vi "NF LI56xx VI Tree.vi"   [LabVIEW 2019]
doc: "The VI Tree displays all the user-callable VIs of the instrument driver in an organized table."
panel:
  # "Copyright(c) 2019 NF Corporation All rights reserved."
  # "SEE DIAGRAM\nFOR VI TREE."
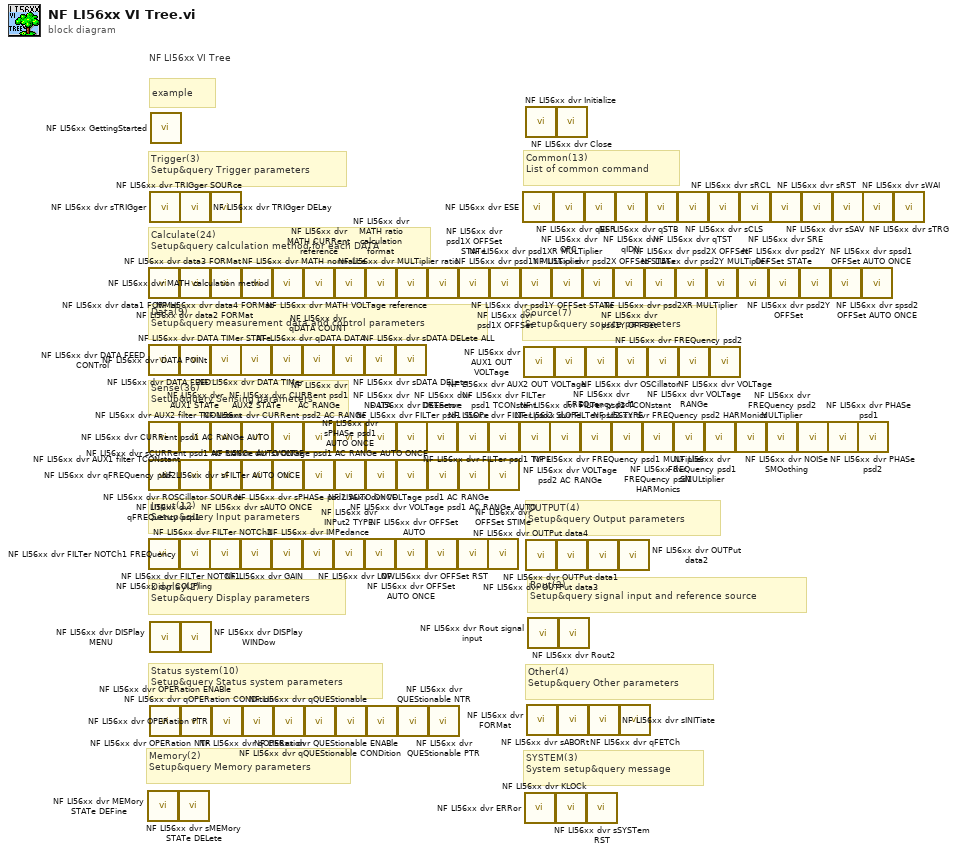
[diagram p0: block diagram]
diagram:
  # "Source(7)\nSetup&query source parameters"
  # "Common(13)\nList of common command"
  # "SYSTEM(3)\nSystem setup&query message"
  # "Memory(2)\nSetup&query Memory parameters"
  # "Status system(10)\nSetup&query Status system parameters"
  # "Other(4)\nSetup&query Other parameters"
  # "OUTPUT(4)\nSetup&query Output parameters"
  # "Input(12)\nSetup&query Input parameters"
  # "Sense(36)\nSetup&query Sensing parameters"
  # "NF LI56xx VI Tree"
  # "Display(2)\nSetup&query Display parameters"
  # "Rout(2)\nSetup&query signal input and reference source"
  # "Calculate(24)\nSetup&query calculation method for each DATA"
  # "Trigger(3)\nSetup&query Trigger parameters"
  # "Data(9)\nSetup&query measurement data and control parameters"
  # "example"
  n1 = call "NF LI56xx dvr MEMory STATe DEFine.vi"() -> ()  [unwired: 9 in, 3 out]
  n2 = call "NF LI56xx dvr data1 FORMat.vi"() -> ()  [unwired: 9 in, 3 out]
  n3 = call "NF LI56xx dvr DATA FEED CONTrol.vi"() -> ()  [unwired: 9 in, 3 out]
  n4 = call "NF LI56xx dvr AUX1 filter TCONstant.vi"() -> ()  [unwired: 9 in, 3 out]
  n5 = call "NF LI56xx dvr qFREQuency psd1.vi"() -> ()  [unwired: 9 in, 3 out]
  n6 = call "NF LI56xx dvr COUPling.vi"() -> ("error out"=w13:errorcluster, "VISA resource name copy"=w12:refnum<visa-resource-name>)  [unwired: 9 in, 1 out]
  n7 = call "NF LI56xx dvr sTRIGger.vi"() -> ("error out"=w4:errorcluster, "VISA resource name copy"=w3:refnum<visa-resource-name>)  [unwired: 10 in]
  n8 = call "NF LI56xx dvr DISPlay MENU.vi"() -> ()  [unwired: 9 in, 3 out]
  n9 = call "NF LI56xx dvr OPERation ENABle.vi"() -> ()  [unwired: 9 in, 3 out]
  n10 = call "NF LI56xx GettingStarted.vi"() -> ()  [unwired: 12 in]
  n11 = call "NF LI56xx dvr sMEMory STATe DELete.vi"() -> ()  [unwired: 10 in, 2 out]
  n12 = call "NF LI56xx dvr TRIGger DELay.vi"() -> ()  [unwired: 9 in, 3 out]
  n13 = call "NF LI56xx dvr data2 FORMat.vi"() -> ()  [unwired: 9 in, 3 out]
  n14 = call "NF LI56xx dvr DATA FEED.vi"() -> ("error out"=w32:errorcluster, "VISA resource name copy"=w31:refnum<visa-resource-name>)  [unwired: 9 in, 1 out]
  n15 = call "NF LI56xx dvr AUX1 STATe.vi"() -> ()  [unwired: 9 in, 3 out]
  n16 = call "NF LI56xx dvr qFREQuency psd2.vi"() -> ()  [unwired: 9 in, 3 out]
  n17 = call "NF LI56xx dvr FILTer NOTCh1 FREQuency.vi"() -> ()  [unwired: 9 in, 3 out]
  n18 = call "NF LI56xx dvr DISPlay WINDow.vi"() -> ()  [unwired: 9 in, 3 out]
  n19 = call "NF LI56xx dvr OPERation NTR.vi"() -> ()  [unwired: 9 in, 3 out]
  n20 = call "NF LI56xx dvr FILTer NOTCh1.vi"("error in"=w13, "VISA resource name"=w12) -> ("error out"=w11:errorcluster, "query notch filter enable"=w10:bool, "VISA resource name copy"=w9:refnum<visa-resource-name>)  [unwired: 7 in]
  n21 = call "NF LI56xx dvr TRIGger SOURce.vi"("error in"=w4, "VISA resource name"=w3) -> ()  [unwired: 7 in, 3 out]
  n22 = call "NF LI56xx dvr data3 FORMat.vi"() -> ()  [unwired: 9 in, 3 out]
  n23 = call "NF LI56xx dvr DATA POINt.vi"() -> ()  [unwired: 9 in, 3 out]
  n24 = call "NF LI56xx dvr AUX2 filter TCONstant.vi"() -> ()  [unwired: 9 in, 3 out]
  n25 = call "NF LI56xx dvr ROSCillator SOURce.vi"() -> ("error out"=w15:errorcluster, "VISA resource name copy"=w14:refnum<visa-resource-name>)  [unwired: 9 in, 1 out]
  n26 = call "NF LI56xx dvr OPERation PTR.vi"() -> ()  [unwired: 9 in, 3 out]
  n27 = call "NF LI56xx dvr DATA TIMer STATe.vi"("error in"=w32, "VISA resource name"=w31) -> ()  [unwired: 7 in, 3 out]
  n28 = call "NF LI56xx dvr FILTer NOTCh2.vi"() -> ()  [unwired: 9 in, 3 out]
  n29 = call "NF LI56xx dvr data4 FORMat.vi"() -> ()  [unwired: 9 in, 3 out]
  n30 = call "NF LI56xx dvr AUX2 STATe.vi"() -> ()  [unwired: 9 in, 3 out]
  n31 = call "NF LI56xx dvr sAUTO ONCE.vi"() -> ()  [unwired: 10 in, 2 out]
  n32 = call "NF LI56xx dvr qOPERation CONDition.vi"() -> ()  [unwired: 9 in, 3 out]
  n33 = call "NF LI56xx dvr DATA TIMer.vi"() -> ()  [unwired: 9 in, 3 out]
  n34 = call "NF LI56xx dvr GAIN.vi"("error in"=w11, "Read(F)"=w10, "VISA resource name"=w9) -> ()  [unwired: 6 in, 3 out]
  n35 = call "NF LI56xx dvr MATH calculation method.vi"() -> ()  [unwired: 9 in, 3 out]
  n36 = call "NF LI56xx dvr CURRent psd1 AC RANGe AUTO.vi"() -> ()  [unwired: 9 in, 3 out]
  n37 = call "NF LI56xx dvr sCURRent psd1 AC RANGe AUTO ONCE.vi"("error in"=w15, "VISA resource name"=w14) -> ()  [unwired: 8 in, 2 out]
  n38 = call "NF LI56xx dvr qOPERation.vi"() -> ()  [unwired: 9 in, 3 out]
  n39 = call "NF LI56xx dvr qDATA COUNT.vi"() -> ()  [unwired: 9 in, 3 out]
  n40 = call "NF LI56xx dvr IMPedance.vi"() -> ()  [unwired: 9 in, 3 out]
  n41 = call "NF LI56xx dvr MATH CURRent reference.vi"() -> ()  [unwired: 9 in, 3 out]
  n42 = call "NF LI56xx dvr CURRent psd1 AC RANGe.vi"() -> ()  [unwired: 9 in, 3 out]
  n43 = call "NF LI56xx dvr sFILTer AUTO ONCE.vi"() -> ()  [unwired: 10 in, 2 out]
  n44 = call "NF LI56xx dvr qQUEStionable CONDition.vi"() -> ()  [unwired: 9 in, 3 out]
  n45 = call "NF LI56xx dvr qDATA DATA.vi"() -> ()  [unwired: 10 in, 2 out]
  n46 = call "NF LI56xx dvr INPut2 TYPE.vi"() -> ()  [unwired: 9 in, 3 out]
  n47 = call "NF LI56xx dvr MATH normalize.vi"() -> ()  [unwired: 9 in, 3 out]
  n48 = call "NF LI56xx dvr CURRent psd2 AC RANGe.vi"() -> ()  [unwired: 9 in, 3 out]
  n49 = call "NF LI56xx dvr sPHASe psd1 AUTO ONCE.vi"() -> ()  [unwired: 10 in, 2 out]
  n50 = call "NF LI56xx dvr qQUEStionable.vi"() -> ()  [unwired: 9 in, 3 out]
  n51 = call "NF LI56xx dvr sDATA DELete ALL.vi"() -> ()  [unwired: 10 in, 2 out]
  n52 = call "NF LI56xx dvr LOW.vi"() -> ()  [unwired: 9 in, 3 out]
  n53 = call "NF LI56xx dvr MATH ratio calculation format.vi"() -> ()  [unwired: 9 in, 3 out]
  n54 = call "NF LI56xx dvr DATA.vi"() -> ("error out"=w30:errorcluster, "VISA resource name copy"=w29:refnum<visa-resource-name>)  [unwired: 9 in, 1 out]
  n55 = call "NF LI56xx dvr sPHASe psd2 AUTO ONCE.vi"() -> ()  [unwired: 10 in, 2 out]
  n56 = call "NF LI56xx dvr QUEStionable ENABle.vi"() -> ()  [unwired: 9 in, 3 out]
  n57 = call "NF LI56xx dvr sDATA DELete.vi"() -> ()  [unwired: 10 in, 2 out]
  n58 = call "NF LI56xx dvr OFFSet AUTO ONCE.vi"() -> ()  [unwired: 10 in, 2 out]
  n59 = call "NF LI56xx dvr MATH VOLTage reference.vi"() -> ()  [unwired: 9 in, 3 out]
  n60 = call "NF LI56xx dvr DETector.vi"() -> ("error out"=w28:errorcluster, "VISA resource name copy"=w27:refnum<visa-resource-name>)  [unwired: 9 in, 1 out]
  n61 = call "NF LI56xx dvr sVOLTage psd1 AC RANGe AUTO ONCE.vi"() -> ()  [unwired: 10 in, 2 out]
  n62 = call "NF LI56xx dvr QUEStionable NTR.vi"() -> ()  [unwired: 9 in, 3 out]
  n63 = call "NF LI56xx dvr DREServe.vi"("error in"=w30, "VISA resource name"=w29) -> ()  [unwired: 7 in, 3 out]
  n64 = call "NF LI56xx dvr OFFSet AUTO.vi"() -> ()  [unwired: 9 in, 3 out]
  n65 = call "NF LI56xx dvr MULTiplier ratio.vi"() -> ()  [unwired: 9 in, 3 out]
  n66 = call "NF LI56xx dvr VOLTage psd1 AC RANGe AUTO.vi"() -> ("error out"=w18:errorcluster, "query AC range \nauto"=w17:bool, "VISA resource name copy"=w16:refnum<visa-resource-name>)  [unwired: 9 in]
  n67 = call "NF LI56xx dvr QUEStionable PTR.vi"() -> ()  [unwired: 9 in, 3 out]
  n68 = call "NF LI56xx dvr FILTer psd1 SLOPe.vi"("error in"=w28, "VISA resource name"=w27) -> ()  [unwired: 7 in, 3 out]
  n69 = call "NF LI56xx dvr OFFSet RST.vi"() -> ()  [unwired: 10 in, 2 out]
  n70 = call "NF LI56xx dvr psd1X OFFSet STATe.vi"() -> ()  [unwired: 9 in, 3 out]
  n71 = call "NF LI56xx dvr VOLTage psd1 AC RANGe.vi"() -> ()  [unwired: 9 in, 3 out]
  n72 = call "NF LI56xx dvr OFFSet STIMe.vi"() -> ()  [unwired: 9 in, 3 out]
  n73 = call "NF LI56xx dvr FILTer psd1 TCONstant.vi"() -> ("error out"=w26:errorcluster, "VISA resource name copy"=w25:refnum<visa-resource-name>)  [unwired: 9 in, 1 out]
  n74 = call "NF LI56xx dvr VOLTage psd2 AC RANGe.vi"("error in"=w18, "Read(F)"=w17, "VISA resource name"=w16) -> ()  [unwired: 6 in, 3 out]
  n75 = call "NF LI56xx dvr psd1X OFFSet.vi"() -> ()  [unwired: 9 in, 3 out]
  n76 = call "NF LI56xx dvr FILTer psd1 TYPE.vi"() -> ("error out"=w24:errorcluster, "VISA resource name copy"=w23:refnum<visa-resource-name>)  [unwired: 9 in, 1 out]
  n77 = call "NF LI56xx dvr psd1XR MULTiplier.vi"() -> ()  [unwired: 9 in, 3 out]
  n78 = call "NF LI56xx dvr ESE.vi"() -> ()  [unwired: 9 in, 3 out]
  n79 = call "NF LI56xx dvr AUX1 OUT VOLTage.vi"() -> ()  [unwired: 9 in, 3 out]
  n80 = call "NF LI56xx dvr ERRor.vi"() -> ()  [unwired: 12 in, 4 out]
  n81 = call "NF LI56xx dvr Initialize.vi"() -> ()  [unwired: 9 in, 3 out]
  n82 = call "NF LI56xx dvr OUTPut data3.vi"() -> ()  [unwired: 9 in, 3 out]
  n83 = call "NF LI56xx dvr FORMat.vi"() -> ()  [unwired: 9 in, 3 out]
  n84 = call "NF LI56xx dvr Rout signal input.vi"() -> ()  [unwired: 9 in, 3 out]
  n85 = call "NF LI56xx dvr FILTer psd2 SLOPe.vi"("error in"=w26, "VISA resource name"=w25) -> ()  [unwired: 7 in, 3 out]
  n86 = call "NF LI56xx dvr psd1Y MULTiplier.vi"() -> ()  [unwired: 9 in, 3 out]
  n87 = call "NF LI56xx dvr OPC.vi"() -> ()  [unwired: 10 in, 2 out]
  n88 = call "NF LI56xx dvr AUX2 OUT VOLTage.vi"() -> ()  [unwired: 9 in, 3 out]
  n89 = call "NF LI56xx dvr KLOCk.vi"() -> ()  [unwired: 9 in, 3 out]
  n90 = call "NF LI56xx dvr Close.vi"() -> ()  [unwired: 10 in, 2 out]
  n91 = call "NF LI56xx dvr OUTPut data4.vi"() -> ()  [unwired: 9 in, 3 out]
  n92 = call "NF LI56xx dvr sABORt.vi"() -> ("error out"=w2:errorcluster, "VISA resource name copy"=w1:refnum<visa-resource-name>)  [unwired: 10 in]
  n93 = call "NF LI56xx dvr Rout2.vi"() -> ()  [unwired: 9 in, 3 out]
  n94 = call "NF LI56xx dvr FILTer psd2 TCONstant.vi"("error in"=w24, "VISA resource name"=w23) -> ()  [unwired: 7 in, 3 out]
  n95 = call "NF LI56xx dvr psd1Y OFFSet STATe.vi"() -> ()  [unwired: 9 in, 3 out]
  n96 = call "NF LI56xx dvr qESR.vi"() -> ()  [unwired: 9 in, 3 out]
  n97 = call "NF LI56xx dvr FREQuency psd1.vi"() -> ()  [unwired: 9 in, 3 out]
  n98 = call "NF LI56xx dvr sSYSTem RST.vi"() -> ()  [unwired: 10 in, 2 out]
  n99 = call "NF LI56xx dvr OUTPut data1.vi"() -> ()  [unwired: 9 in, 3 out]
  n100 = call "NF LI56xx dvr sINITiate.vi"() -> ()  [unwired: 10 in, 2 out]
  n101 = call "NF LI56xx dvr FILTer psd2 TYPE.vi"() -> ()  [unwired: 9 in, 3 out]
  n102 = call "NF LI56xx dvr psd1Y OFFSet.vi"() -> ()  [unwired: 9 in, 3 out]
  n103 = call "NF LI56xx dvr qIDN.vi"() -> ()  [unwired: 9 in, 3 out]
  n104 = call "NF LI56xx dvr FREQuency psd2.vi"() -> ()  [unwired: 9 in, 3 out]
  n105 = call "NF LI56xx dvr OUTPut data2.vi"() -> ()  [unwired: 9 in, 3 out]
  n106 = call "NF LI56xx dvr qFETCh.vi"("error in"=w2, "VISA resource name"=w1) -> ()  [unwired: 7 in, 3 out]
  n107 = call "NF LI56xx dvr FREQuency psd1 HARMonics.vi"() -> ()  [unwired: 9 in, 3 out]
  n108 = call "NF LI56xx dvr psd2X OFFSet STATe.vi"() -> ()  [unwired: 9 in, 3 out]
  n109 = call "NF LI56xx dvr qSTB.vi"() -> ()  [unwired: 9 in, 3 out]
  n110 = call "NF LI56xx dvr OSCillator.vi"() -> ()  [unwired: 9 in, 3 out]
  n111 = call "NF LI56xx dvr FREQuency psd1 MULTiplier.vi"() -> ()  [unwired: 9 in, 3 out]
  n112 = call "NF LI56xx dvr psd2X OFFSet.vi"() -> ()  [unwired: 9 in, 3 out]
  n113 = call "NF LI56xx dvr qTST.vi"() -> ()  [unwired: 9 in, 3 out]
  n114 = call "NF LI56xx dvr VOLTage RANGe.vi"() -> ()  [unwired: 9 in, 3 out]
  n115 = call "NF LI56xx dvr FREQuency psd1 SMULtiplier.vi"() -> ()  [unwired: 9 in, 3 out]
  n116 = call "NF LI56xx dvr psd2XR MULTiplier.vi"() -> ()  [unwired: 9 in, 3 out]
  n117 = call "NF LI56xx dvr sCLS.vi"() -> ()  [unwired: 10 in, 2 out]
  n118 = call "NF LI56xx dvr VOLTage.vi"() -> ()  [unwired: 9 in, 3 out]
  n119 = call "NF LI56xx dvr FREQuency psd2 HARMonics.vi"() -> ()  [unwired: 9 in, 3 out]
  n120 = call "NF LI56xx dvr psd2Y MULTiplier.vi"() -> ()  [unwired: 9 in, 3 out]
  n121 = call "NF LI56xx dvr sRCL.vi"() -> ()  [unwired: 10 in, 2 out]
  n122 = call "NF LI56xx dvr FREQuency psd2 MULTiplier.vi"() -> ("error out"=w22:errorcluster, "VISA resource name copy"=w21:refnum<visa-resource-name>)  [unwired: 9 in, 1 out]
  n123 = call "NF LI56xx dvr psd2Y OFFSet STATe.vi"() -> ()  [unwired: 9 in, 3 out]
  n124 = call "NF LI56xx dvr SRE.vi"() -> ()  [unwired: 9 in, 3 out]
  n125 = call "NF LI56xx dvr NOISe SMOothing.vi"() -> ("error out"=w20:errorcluster, "VISA resource name copy"=w19:refnum<visa-resource-name>)  [unwired: 9 in, 1 out]
  n126 = call "NF LI56xx dvr psd2Y OFFSet.vi"() -> ()  [unwired: 9 in, 3 out]
  n127 = call "NF LI56xx dvr sRST.vi"() -> ("error out"=w8:errorcluster, "VISA resource name copy"=w7:refnum<visa-resource-name>)  [unwired: 10 in]
  n128 = call "NF LI56xx dvr PHASe psd1.vi"("error in"=w22, "VISA resource name"=w21) -> ()  [unwired: 7 in, 3 out]
  n129 = call "NF LI56xx dvr spsd1 OFFSet AUTO ONCE.vi"() -> ()  [unwired: 10 in, 2 out]
  n130 = call "NF LI56xx dvr sSAV.vi"() -> ("error out"=w6:errorcluster, "VISA resource name copy"=w5:refnum<visa-resource-name>)  [unwired: 10 in]
  n131 = call "NF LI56xx dvr PHASe psd2.vi"("error in"=w20, "VISA resource name"=w19) -> ()  [unwired: 7 in, 3 out]
  n132 = call "NF LI56xx dvr spsd2 OFFSet AUTO ONCE.vi"() -> ()  [unwired: 10 in, 2 out]
  n133 = call "NF LI56xx dvr sWAI.vi"("error in"=w8, "VISA resource name"=w7) -> ()  [unwired: 8 in, 2 out]
  n134 = call "NF LI56xx dvr sTRG.vi"("error in"=w6, "VISA resource name"=w5) -> ()  [unwired: 8 in, 2 out]
